vi "FindMiddlePoint.vi"(3 "left":i16, 5 "right":i16) -> (1 "middle":dbl)   [LabVIEW 2022 SP3]
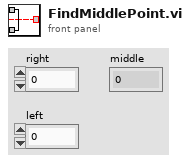
[diagram p1: front panel]
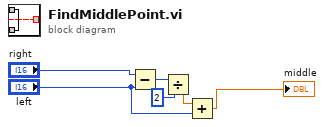
[diagram p0: block diagram]
diagram:
  n1 = Subtract(x="right", y="left") -> (x-y=w2:i16)
  n2 = Divide(x=w2, y=i16 2) -> (x/y=w5:dbl)
  n3 = Add(x=w5, y="left") -> (x+y=→"middle":dbl)
